vi "MsgPack.vi"(8 "error in":errorcluster, 9 "msg":string, 10 "msg_id":u16, 11 "msg_type":T1=enum."LOGIN") -> (0 "error out":errorcluster, 2 "msg_data":string)   [LabVIEW 2014]
uses:
  MsgType.ctl
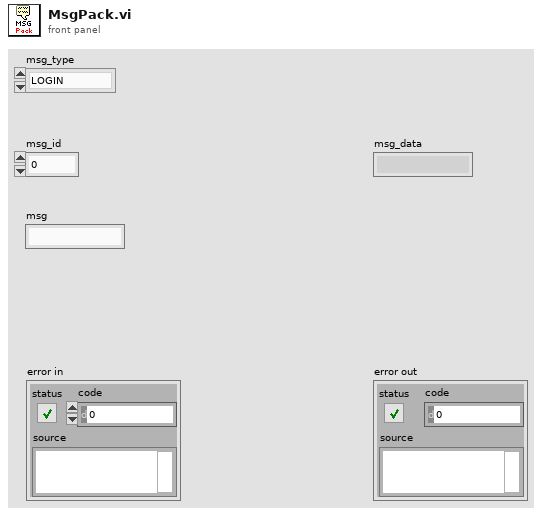
[diagram p1: front panel]
types:
  T1 = typedef "MsgType.ctl" = enum8{"RSP", "REGISTER", "LOGIN", "SAVE_PROF", "LOAD_PROF", "GET_TOKEN", "PING", "ACTIVATE", "DEACTIVATE", "REFRESH", "UNDEFINED0", "UNDEFINED1", "TWEET", "EMAIL", "NOTIFY", "BRIDGE", "UNDEFINED2", "UNDEFINED3", "UNDEFINED4", "UNDEFINED5", "HW"}
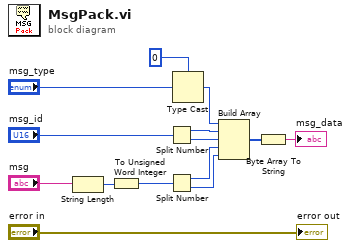
[diagram p0: block diagram]
diagram:
  n1 = String Length(string="msg") -> (length=w14:i32)
  n2 = To Unsigned Word Integer(number=w14) -> (unsigned 16bit integer=w12:u16)
  n3 = Split Number(x="msg_id") -> (hi(x)=w8:u8, lo(x)=w13:u8)
  n4 = Split Number(x=w12) -> (hi(x)=w11:u8, lo(x)=w10:u8)
  n5 = Type Cast(type=u8 0, x="msg_type") -> (*(type *) &x=w6:u8)
  n6 = Build Array(w6, w8, w13, w11, w10) -> (w9:u8[])
  n7 = Byte Array To String(unsigned byte array=w9) -> (string=→"msg_data":string)
  "error out" <- "error in"
